vi "DHE_GetExtShutter.vi"() -> (7 "Ext_Shutter":bool)   [LabVIEW 2016]
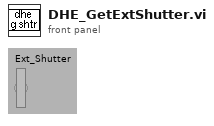
[diagram p1: front panel]
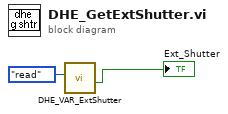
[diagram p0: block diagram]
diagram:
  n1 = call "DHE_VAR_ExtShutter.vi"("action"=enum16{"read", "write"}."read") -> ("external shutter?"=→"Ext_Shutter":bool)  [unwired: 1 in, 9 out]
